vi "EnableDisapleControlls_ELOGTab.vi"(7 "Enum":enum16{"StartBuffer", "StopBuffer"}(ring)=enum."StopBuffer", 8 "error in (no error)":errorcluster, 11 "Common Refs":T1={"LBox_ChList"=refnum, "STR_LoggingChName1"=refnum, "Listbox_ChValue"=refnum, "STR_LoggingChName2"=refnum, "STR_LoggingChName3"=refnum, "STR_LoggingChName4"=refnum, "STR_LoggingChName5"=refnum, "STR_LoggingChName6"=refnum, "OXY_SCPI Ref"="TCPIP0::192.168.1.75::10001::SOCKET", "STR_ChName1"=refnum, "STR_ChName2"=refnum, "STR_ChName3"=refnum, "STR_ChName4"=refnum, "STR_ChName5"=refnum, "STR_ChName6"=refnum, "Enum_SelectTimestampFormat"=refnum, "GRAPH-XY_ELOG"=refnum, "GRAPH-XY_Measurement"=refnum, "Button_StartBuffer"=refnum, "Button_StopBuffer"=refnum, "Button_FetchData"=refnum, "STR_LoggingChName1"=refnum, "STR_LoggingChName2"=refnum, "STR_LoggingChName3"=refnum, "STR_LoggingChName4"=refnum, "STR_LoggingChName5"=refnum, "STR_LoggingChName6"=refnum, "Enum_SelectCalc"=refnum, "Num_SetDurationTime"=refnum, "Button_StopTransfer"=refnum, "Button_StartTransfer"=refnum, "STR_IN_AggregationRate"=refnum, "Button_Disconnect"=refnum, "Button_Connect"=refnum, "Button_StartRec"=refnum, "Button_PauseRec"=refnum, "Button_StopRec"=refnum, "Bool_StatusLED"=refnum, "Indicator_RecordingStatus"=refnum}) -> (0 "error out":errorcluster)   [LabVIEW 2018]
uses:
  TypeDefs/Refs_Common.ctl
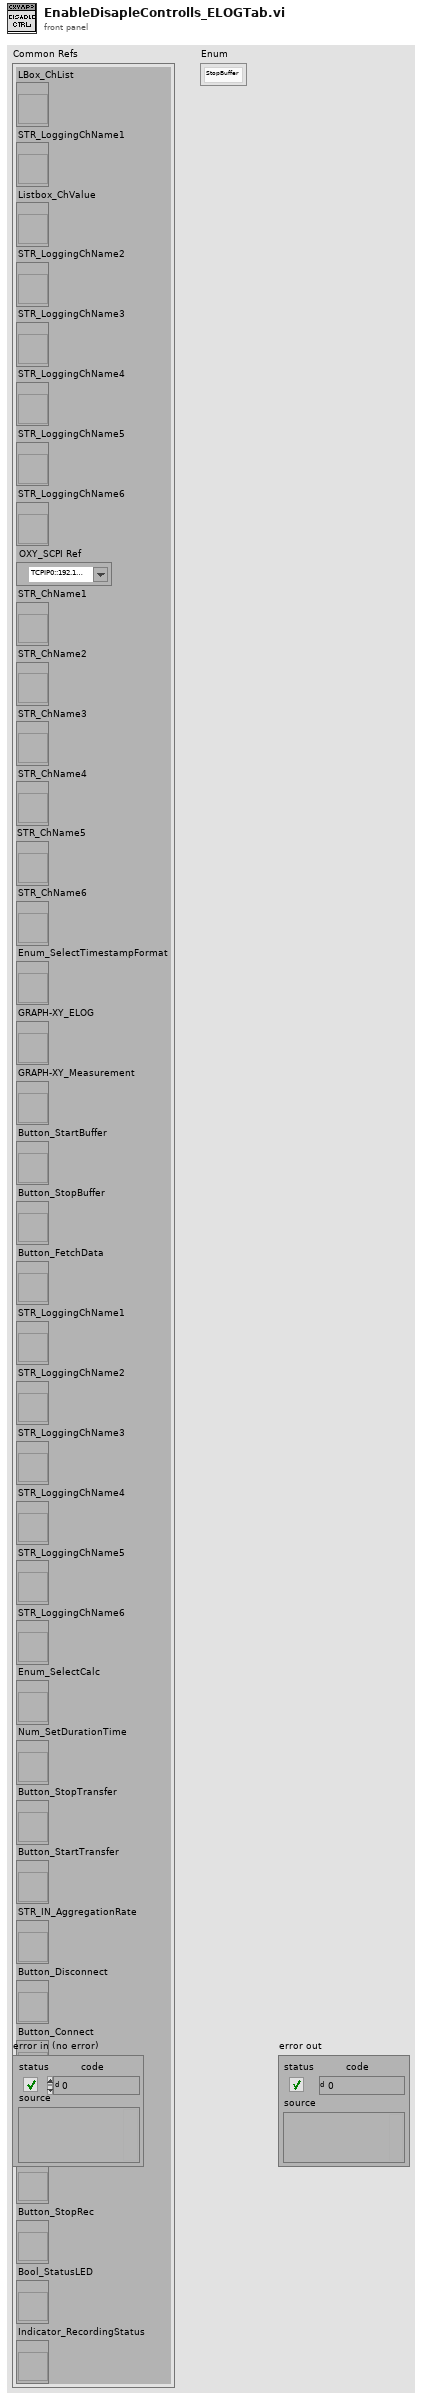
[diagram p1: front panel]
types:
  T1 = typedef "Refs_Common.ctl" = cluster{"LBox_ChList":refnum<vi>, "STR_LoggingChName1":refnum<vi>, "Listbox_ChValue":refnum<vi>, "STR_LoggingChName2":refnum<vi>, "STR_LoggingChName3":refnum<vi>, "STR_LoggingChName4":refnum<vi>, "STR_LoggingChName5":refnum<vi>, "STR_LoggingChName6":refnum<vi>, "OXY_SCPI Ref":refnum<visa-resource-name>, "STR_ChName1":refnum<vi>, "STR_ChName2":refnum<vi>, "STR_ChName3":refnum<vi>, "STR_ChName4":refnum<vi>, "STR_ChName5":refnum<vi>, "STR_ChName6":refnum<vi>, "Enum_SelectTimestampFormat":refnum<vi>, "GRAPH-XY_ELOG":refnum<vi>, "GRAPH-XY_Measurement":refnum<vi>, "Button_StartBuffer":refnum<vi>, "Button_StopBuffer":refnum<vi>, "Button_FetchData":refnum<vi>, "STR_LoggingChName1":refnum<vi>, "STR_LoggingChName2":refnum<vi>, "STR_LoggingChName3":refnum<vi>, "STR_LoggingChName4":refnum<vi>, "STR_LoggingChName5":refnum<vi>, "STR_LoggingChName6":refnum<vi>, "Enum_SelectCalc":refnum<vi>, "Num_SetDurationTime":refnum<vi>, "Button_StopTransfer":refnum<vi>, "Button_StartTransfer":refnum<vi>, "STR_IN_AggregationRate":refnum<vi>, "Button_Disconnect":refnum<vi>, "Button_Connect":refnum<vi>, "Button_StartRec":refnum<vi>, "Button_PauseRec":refnum<vi>, "Button_StopRec":refnum<vi>, "Bool_StatusLED":refnum<vi>, "Indicator_RecordingStatus":refnum<vi>}
  T2 = enum8{"Enabled", "Disabled", "Disabled and Grayed Out"}
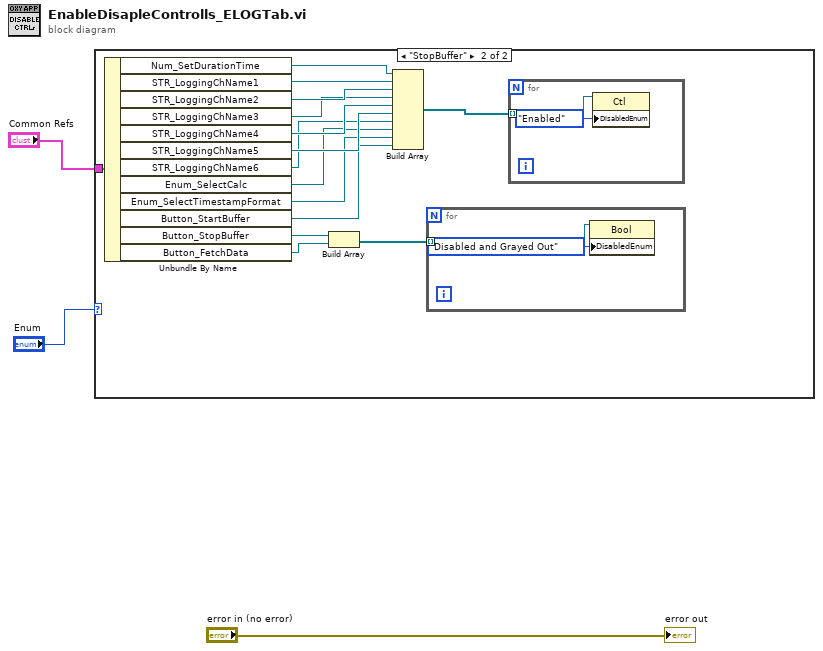
[diagram p0: block diagram]
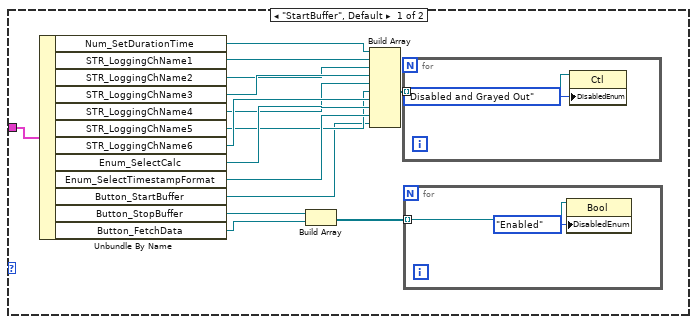
[diagram p2: hidden frame]
diagram:
  n1 = case shown="\"StopBuffer\"" "Enum" {
    tunnel: "Common Refs" -> [w7 w37]
    frame "StartBuffer", Default {
      n2 = Unbundle By Name(w7) -> ("Num_SetDurationTime"=w4:refnum<vi>, "STR_LoggingChName1"=w8:refnum<vi>, "STR_LoggingChName2"=w9:refnum<vi>, "STR_LoggingChName3"=w10:refnum<vi>, "STR_LoggingChName4"=w11:refnum<vi>, "STR_LoggingChName5"=w6:refnum<vi>, "STR_LoggingChName6"=w12:refnum<vi>, "Enum_SelectCalc"=w13:refnum<vi>, "Enum_SelectTimestampFormat"=w14:refnum<vi>, "Button_StartBuffer"=w5:refnum<vi>, "Button_StopBuffer"=w16:refnum<vi>, "Button_FetchData"=w17:refnum<vi>)
      n3 = Build Array(w16, w17) -> (w18:refnum<vi>[])
      n4 = Build Array(w4, w8, w9, w10, w11, w6, w12, w13, w14, w5) -> (w15:refnum<vi>[])
      n5 = for {
        tunnel: w15 -> [w22] mode=indexing
        n6 = property class="Ctl"(reference=w22, "DisabledEnum"=T2."Disabled and Grayed Out" ("Disabled")) -> ()  [unwired: 1 in, 2 out]
      }
      n7 = for {
        tunnel: w18 -> [w20] mode=indexing
        n8 = property class="Bool"(reference=w20, "DisabledEnum"=T2."Enabled" ("Disabled")) -> ()  [unwired: 1 in, 2 out]
      }
    }
    frame "StopBuffer" {
      n9 = Unbundle By Name(w37) -> ("Num_SetDurationTime"=w23:refnum<vi>, "STR_LoggingChName1"=w36:refnum<vi>, "STR_LoggingChName2"=w35:refnum<vi>, "STR_LoggingChName3"=w34:refnum<vi>, "STR_LoggingChName4"=w33:refnum<vi>, "STR_LoggingChName5"=w32:refnum<vi>, "STR_LoggingChName6"=w31:refnum<vi>, "Enum_SelectCalc"=w30:refnum<vi>, "Enum_SelectTimestampFormat"=w29:refnum<vi>, "Button_StartBuffer"=w28:refnum<vi>, "Button_StopBuffer"=w26:refnum<vi>, "Button_FetchData"=w25:refnum<vi>)
      n10 = Build Array(w26, w25) -> (w24:refnum<vi>[])
      n11 = Build Array(w23, w36, w35, w34, w33, w32, w31, w30, w29, w28) -> (w27:refnum<vi>[])
      n12 = for {
        tunnel: w24 -> [w39] mode=indexing
        n13 = property class="Bool"(reference=w39, "DisabledEnum"=T2."Disabled and Grayed Out" ("Disabled")) -> ()  [unwired: 1 in, 2 out]
      }
      n14 = for {
        tunnel: w27 -> [w41] mode=indexing
        n15 = property class="Ctl"(reference=w41, "DisabledEnum"=T2."Enabled" ("Disabled")) -> ()  [unwired: 1 in, 2 out]
      }
    }
  }
  "error out" <- "error in (no error)"
